vi "Log Error.vi"(10 "error in (no error)":errorcluster, 11 "SOL-Server in":refnum<class "SOL-Server.lvclass">) -> (3 "SOL-Server out":refnum<class "SOL-Server.lvclass">)   [LabVIEW 2020, in "Summer of LabVIEW.lvlib" / "SOL-Server.lvclass"]
uses:
  SOL-Server.lvclass
  SOL-Server.lvclass/SOL-Server.ctl
  Error Log.ctl
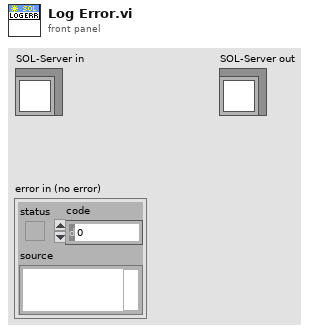
[diagram p1: front panel]
types:
  T1 = typedef "Summer of LabVIEW.lvlib/SOL-Server.lvclass/Error Log.ctl" = cluster{"Time Stamp":timestamp, "Code":i32, "Source":string}
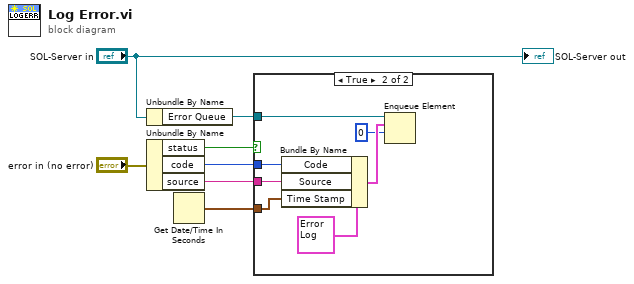
[diagram p0: block diagram]
diagram:
  n1 = Unbundle By Name("SOL-Server in") -> ("Error Queue"=w4:refnum<queue>)
  n2 = Unbundle By Name("error in (no error)") -> ("status"=w6:bool, "code"=w3:i32, "source"=w2:string)
  n3 = Get Date/Time In Seconds() -> (seconds since 1Jan1904=w1:timestamp)
  n4 = case shown="True" w6 {
    tunnel: w4 -> [_ w10]
    tunnel: w3 -> [_ w13]
    tunnel: w2 -> [_ w12]
    tunnel: w1 -> [_ w11]
    frame False {
    }
    frame True {
      n5 = Bundle By Name(cluster=T1 {"Time Stamp"=timestamp(0 s since 1904-01-01), "Code"=0, "Source"=""} ("Error Log"), "Code"=w13, "Source"=w12, "Time Stamp"=w11) -> (w9:T1)
      n6 = Enqueue Element(queue=w10, element=w9, timeout in ms (-1)=0) -> ()  [unwired: 1 in, 3 out]
    }
  }
  "SOL-Server out" <- "SOL-Server in"
